vi "OszilloscopeInit.vi"(8 "Error_in":errorcluster, 11 "VISA Name OZ in(OZ)":refnum<visa-resource-name>="USB0::0x0957::0x179B::MY54313507::INSTR") -> (0 "Error_out":errorcluster)   [LabVIEW 2016]
doc: "Mit diesem VI wird das Oszilloscope DSO-X-2002A initialisiert."
uses:
  <instrlib>/Agilent 2000 3000 X-Series/Agilent 2000 3000 X-Series.lvlib
panel:
  in  "Vertikale Skalierung (0,015 V/div)":dbl=0.015
  in  "Zeit Skalierung (0.004 Sec/div)":dbl=0.004
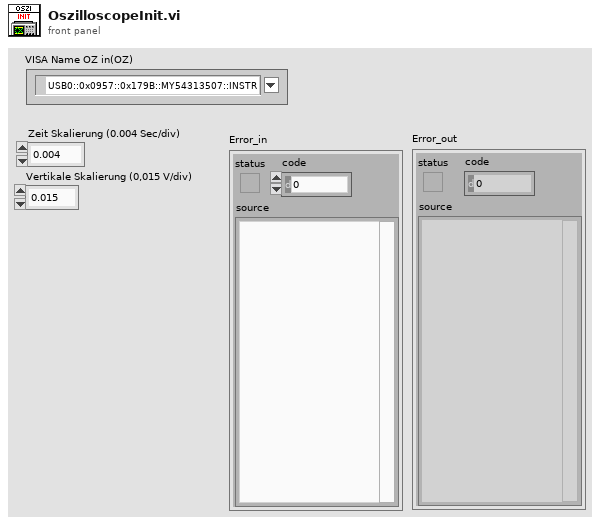
[diagram p1: front panel]
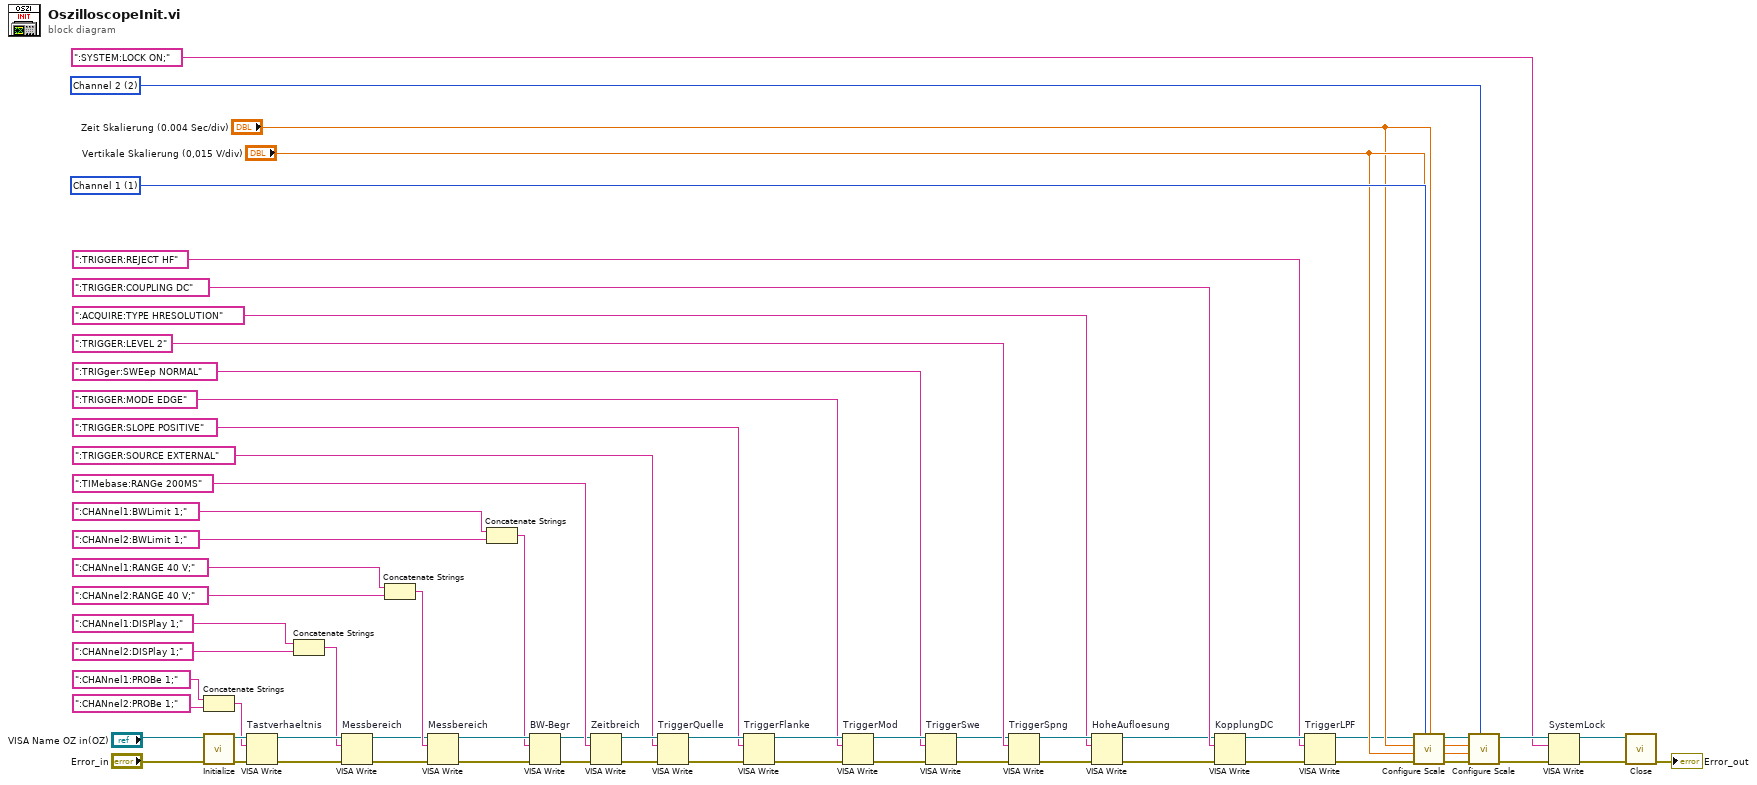
[diagram p0: block diagram]
diagram:
  w42 = 2 items=["Channel 1"=1, "Channel 2"=2, "Channel 3"=3, "Channel 4"=4] ("Channel Name (1: Channel 1)")
  w63 = 1 items=["Channel 1"=1, "Channel 2"=2, "Channel 3"=3, "Channel 4"=4] ("Channel Name (1: Channel 1)")
  n1 = Concatenate Strings(":CHANnel1:PROBe 1;" ("Schreibpuffer"), ":CHANnel2:PROBe 1;" ("Schreibpuffer")) -> (w47:string)
  n2 = call <instrlib>:"Initialize.vi"("error in (no error)"="Error_in", "VISA resource name"="VISA Name OZ in(OZ)") -> ("error out"=w59:errorcluster, "VISA resource name out"=w60:refnum<visa-resource-name>)  [unwired: 8 in]
  n3 = VISA Write "Tastverhaeltnis"(VISA resource name=w60, write buffer=w47, error in (no error)=w59) -> (VISA resource name out=w7:refnum<visa-resource-name>, error out=w5:errorcluster)  [unwired: 1 out]
  n4 = Concatenate Strings(":CHANnel1:DISPlay 1;" ("Schreibpuffer"), ":CHANnel2:DISPlay 1;" ("Schreibpuffer")) -> (w1:string)
  n5 = VISA Write "Messbereich"(VISA resource name=w7, write buffer=w1, error in (no error)=w5) -> (VISA resource name out=w6:refnum<visa-resource-name>, error out=w4:errorcluster)  [unwired: 1 out]
  n6 = Concatenate Strings(":CHANnel1:RANGE 40 V;" ("Schreibpuffer"), ":CHANnel2:RANGE 40 V;" ("Schreibpuffer")) -> (w52:string)
  n7 = VISA Write "Messbereich"(VISA resource name=w6, write buffer=w52, error in (no error)=w4) -> (VISA resource name out=w57:refnum<visa-resource-name>, error out=w56:errorcluster)  [unwired: 1 out]
  n8 = Concatenate Strings(":CHANnel1:BWLimit 1;" ("Schreibpuffer"), ":CHANnel2:BWLimit 1;" ("Schreibpuffer")) -> (w53:string)
  n9 = VISA Write "BW-Begr"(VISA resource name=w57, write buffer=w53, error in (no error)=w56) -> (VISA resource name out=w41:refnum<visa-resource-name>, error out=w40:errorcluster)  [unwired: 1 out]
  n10 = VISA Write "Zeitbreich"(VISA resource name=w41, write buffer=":TIMebase:RANGe 200MS" ("Schreibpuffer"), error in (no error)=w40) -> (VISA resource name out=w35:refnum<visa-resource-name>, error out=w34:errorcluster)  [unwired: 1 out]
  n11 = VISA Write "TriggerQuelle"(VISA resource name=w35, write buffer=":TRIGGER:SOURCE EXTERNAL" ("Schreibpuffer"), error in (no error)=w34) -> (VISA resource name out=w39:refnum<visa-resource-name>, error out=w38:errorcluster)  [unwired: 1 out]
  n12 = VISA Write "TriggerFlanke"(VISA resource name=w39, write buffer=":TRIGGER:SLOPE POSITIVE" ("Schreibpuffer"), error in (no error)=w38) -> (VISA resource name out=w37:refnum<visa-resource-name>, error out=w36:errorcluster)  [unwired: 1 out]
  n13 = VISA Write "TriggerMod"(VISA resource name=w37, write buffer=":TRIGGER:MODE EDGE" ("Schreibpuffer"), error in (no error)=w36) -> (VISA resource name out=w25:refnum<visa-resource-name>, error out=w24:errorcluster)  [unwired: 1 out]
  n14 = VISA Write "TriggerSwe"(VISA resource name=w25, write buffer=":TRIGger:SWEep NORMAL" ("Schreibpuffer"), error in (no error)=w24) -> (VISA resource name out=w23:refnum<visa-resource-name>, error out=w22:errorcluster)  [unwired: 1 out]
  n15 = VISA Write "TriggerSpng"(VISA resource name=w23, write buffer=":TRIGGER:LEVEL 2" ("Schreibpuffer"), error in (no error)=w22) -> (VISA resource name out=w17:refnum<visa-resource-name>, error out=w16:errorcluster)  [unwired: 1 out]
  n16 = VISA Write "HoheAufloesung"(VISA resource name=w17, write buffer=":ACQUIRE:TYPE HRESOLUTION" ("Schreibpuffer"), error in (no error)=w16) -> (VISA resource name out=w15:refnum<visa-resource-name>, error out=w14:errorcluster)  [unwired: 1 out]
  n17 = VISA Write "KopplungDC"(VISA resource name=w15, write buffer=":TRIGGER:COUPLING DC" ("Schreibpuffer"), error in (no error)=w14) -> (VISA resource name out=w32:refnum<visa-resource-name>, error out=w31:errorcluster)  [unwired: 1 out]
  n18 = VISA Write "TriggerLPF"(VISA resource name=w32, write buffer=":TRIGGER:REJECT HF" ("Schreibpuffer"), error in (no error)=w31) -> (VISA resource name out=w19:refnum<visa-resource-name>, error out=w20:errorcluster)  [unwired: 1 out]
  n19 = call <instrlib>:"Configure Scale.vi"("Channel Name (1: Channel 1)"=w63, "error in (no error)"=w20, "Vertical Scale (5 V/div)"="Vertikale Skalierung (0,015 V/div)", "Time Scale (0.0001 Sec/div)"="Zeit Skalierung (0.004 Sec/div)", "VISA resource name"=w19) -> ("error out"=w44:errorcluster, "VISA resource name out"=w43:refnum<visa-resource-name>)  [unwired: 5 in]
  n20 = call <instrlib>:"Configure Scale.vi"("Channel Name (1: Channel 1)"=w42, "error in (no error)"=w44, "Vertical Scale (5 V/div)"="Vertikale Skalierung (0,015 V/div)", "Time Scale (0.0001 Sec/div)"="Zeit Skalierung (0.004 Sec/div)", "VISA resource name"=w43) -> ("error out"=w11:errorcluster, "VISA resource name out"=w12:refnum<visa-resource-name>)  [unwired: 5 in]
  n21 = VISA Write "SystemLock"(VISA resource name=w12, write buffer=":SYSTEM:LOCK ON;", error in (no error)=w11) -> (VISA resource name out=w9:refnum<visa-resource-name>, error out=w10:errorcluster)  [unwired: 1 out]
  n22 = call <instrlib>:"Close.vi"("error in (no error)"=w10, "VISA resource name"=w9) -> ("error out"=→"Error_out":errorcluster)  [unwired: 9 in]
